vi "Get Relay Names.vi"(8 "error in (no error)":errorcluster, 11 "2575 in":refnum<class "2575.lvclass">) -> (0 "error out":errorcluster, 3 "2575 out":refnum<class "2575.lvclass">)   [LabVIEW 2019, in "2575.lvlib" / "2575.lvclass"]
uses:
  Library/2575.lvclass
  Library/2575.lvclass/2575.ctl
  Accessors/Read Local Resource.vi
  Accessors/Write Local Resource.vi
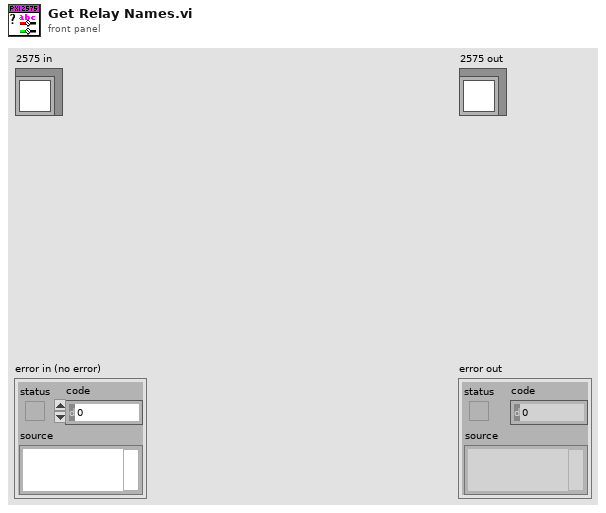
[diagram p1: front panel]
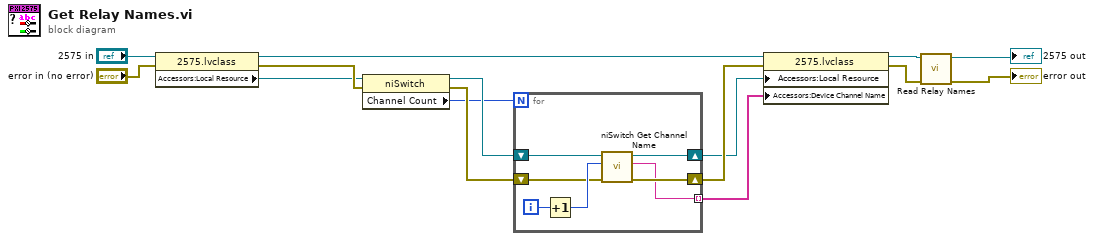
[diagram p0: block diagram]
diagram:
  n1 = property class="2575.lvclass"(reference="2575 in", error in="error in (no error)") -> (reference out=w14:refnum<class "2575.lvclass">, error out=w15:errorcluster, "Accessors:Local Resource"=w13:refnum<k15>)
  n2 = property class="niSwitch"(reference=w13, error in=w15) -> (reference out=w6:refnum<k15>, error out=w8:errorcluster, "Channel Count"=w3:i32)
  n3 = for {
    N: w3 -> [_]
    shift-right: [w18] -> w5
    shift-left: w6 -> [w17]
    shift-right: [w19] -> w7
    shift-left: w8 -> [w20]
    tunnel: [w16] -> w4 mode=indexing
    i -> [w22]
    n4 = Increment(x=w22) -> (x+1=w21:i32)
    n5 = call <instrlib>:"niSwitch Get Channel Name.vi"("error in (no error)"=w20, "index (1)"=w21, "instrument handle"=w17) -> ("error out"=w19:errorcluster, "channel string"=w16:string, "instrument handle out"=w18:refnum<k15>)  [unwired: 6 in]
  }
  n6 = property class="2575.lvclass"(reference=w14, error in=w7, "Accessors:Local Resource"=w5, "Accessors:Device Channel Name"=w4) -> (reference out=w2:refnum<class "2575.lvclass">, error out=w1:errorcluster)
  n7 = call "Read Relay Names.vi"("error in"=w1, "2575 in"=w2) -> ("error out"=→"error out":errorcluster, "2575 out"=→"2575 out":refnum<class "2575.lvclass">)  [unwired: 8 in]
